vi "File_Info.vi"(1 "Path":path, 5 "error in (no error)":errorcluster) -> (14 "LV file?":bool, 15 "LLB?":bool, 16 "Folder?":bool, 17 "Valid path?":bool, 19 "error out":errorcluster)   [LabVIEW 2020]
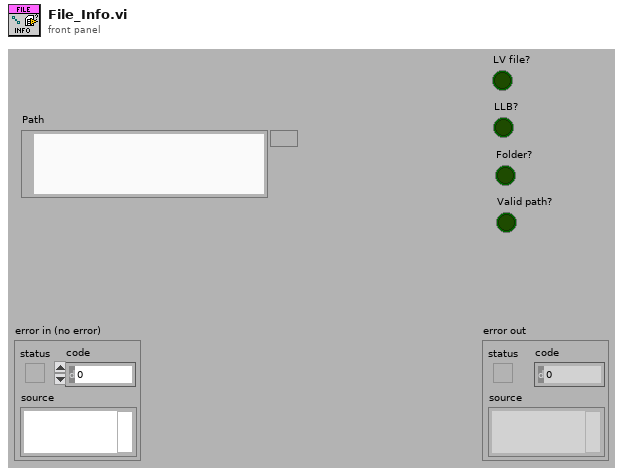
[diagram p1: front panel]
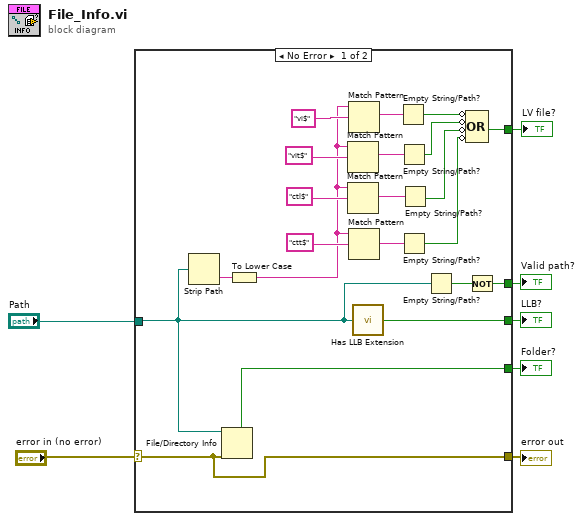
[diagram p0: block diagram]
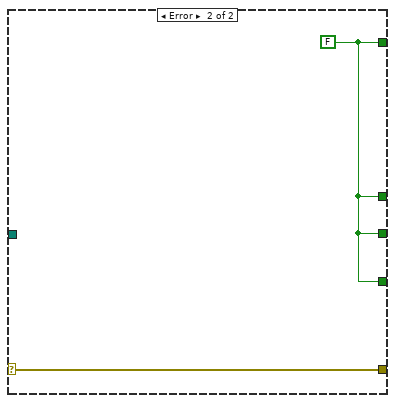
[diagram p2: hidden frame]
diagram:
  n1 = case shown="No Error" "error in (no error)" {
    selector: "error in (no error)" -> [w8 w30]
    tunnel: [w8 w30] -> w6
    tunnel: "Path" -> [w11 _]
    tunnel: [w28 w29] -> w4
    tunnel: [w27 w29] -> w3
    tunnel: [w12 w29] -> w2
    tunnel: [w9 w29] -> w1
    frame No Error {
      n2 = Strip Path(path=w11) -> (name=w26:string)  [unwired: 1 out]
      n3 = File/Directory Info(path=w11, error in=w8) -> (directory=w27:bool)  [unwired: 6 out]
      n4 = To Lower Case(string=w26) -> (all lower case string=w13:string)
      n5 = Match Pattern(string=w13, regular expression="vit$") -> (match substring=w20:string)  [unwired: 4 out]
      n6 = Match Pattern(string=w13, regular expression="ctl$") -> (match substring=w19:string)  [unwired: 4 out]
      n7 = Match Pattern(string=w13, regular expression="vi$") -> (match substring=w21:string)  [unwired: 4 out]
      n8 = Match Pattern(string=w13, regular expression="ctt$") -> (match substring=w18:string)  [unwired: 4 out]
      n9 = call <vilib>:"Has LLB Extension.vi"("path"=w11) -> ("path to VI library?"=w28:bool)
      n10 = Empty String/Path?(string/path=w21) -> (empty?=w17:bool)
      n11 = Empty String/Path?(string/path=w20) -> (empty?=w16:bool)
      n12 = Empty String/Path?(string/path=w18) -> (empty?=w14:bool)
      n13 = Empty String/Path?(string/path=w19) -> (empty?=w15:bool)
      n14 = Empty String/Path?(string/path=w11) -> (empty?=w10:bool)
      n15 = Compound Arithmetic op=OR(invert w17, invert w16, invert w15, invert w14) -> (w12:bool)
      n16 = Not(x=w10) -> (.not. x?=w9:bool)
    }
    frame Error {
      w29 = FALSE
    }
  }
  "error out" <- w6
  "LV file?" <- w2
  "LLB?" <- w4
  "Folder?" <- w3
  "Valid path?" <- w1
